vi "Main2.vi"() -> ()   [LabVIEW 2018]
uses:
  <vilib>/addons/zeromq/zmq_context.lvclass
  Communication Channel/Communication Channel.lvclass
  Channel Rep/Channel Rep.lvclass
  C:/Users/Denis/Desktop/communication-manager/communication-manager/Communication Channel/Communication Channel.lvclass
  Channel Req/Channel Req.lvclass
  Channel Pub/Channel Pub.lvclass
  Channel Sub/Channel Sub.lvclass
panel:
  in  "Channel Pub.lvclass":refnum<class "Channel Pub.lvclass">
  in  "Channel Sub.lvclass":refnum<class "Channel Sub.lvclass">
  in  "Channel Req.lvclass":refnum<class "Channel Req.lvclass">
  in  "Channel Rep.lvclass":refnum<class "Channel Rep.lvclass">
  out "context":refnum<class "zmq_context.lvclass">
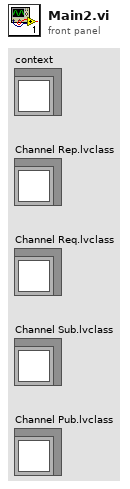
[diagram p1: front panel]
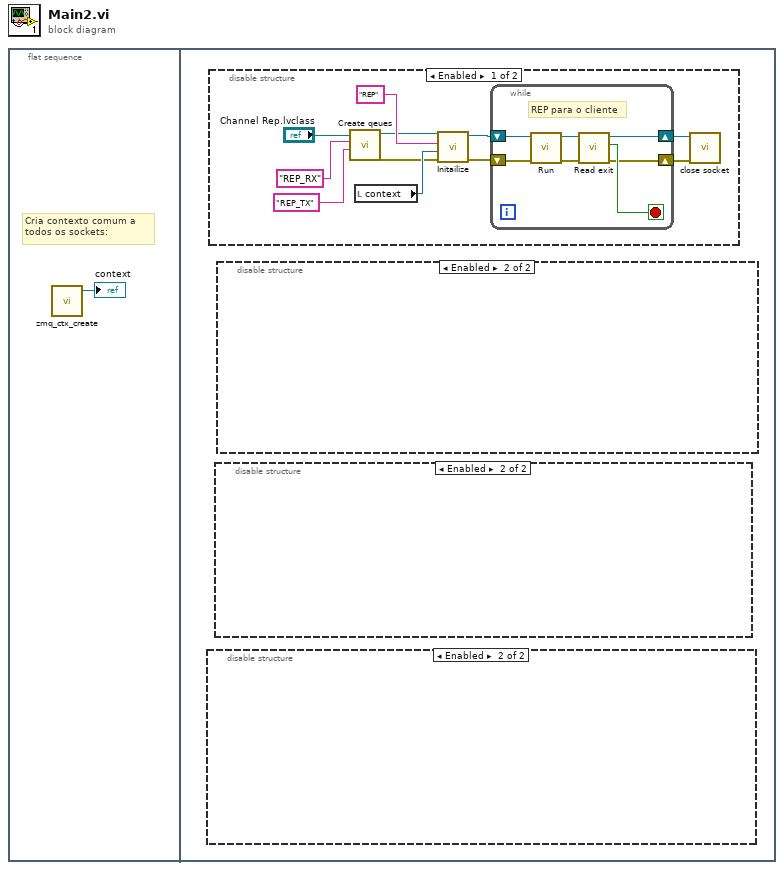
[diagram p0: block diagram]
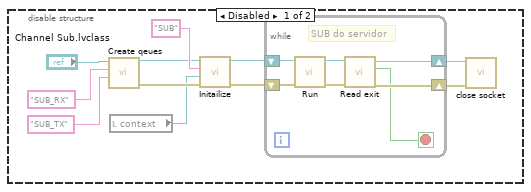
[diagram p2: hidden frame]
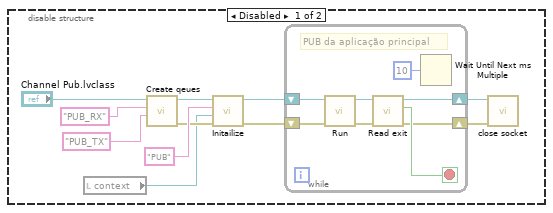
[diagram p3: hidden frame]
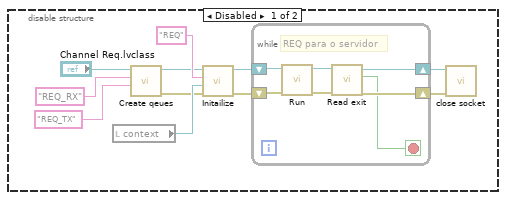
[diagram p4: hidden frame]
diagram:
  n1 = flat-sequence {
    frame #0 {
      # "Cria contexto comum a \ntodos os sockets:"
      n2 = call <vilib>:"zmq_ctx_create.vi"() -> ("context out"=→"context":refnum<class "zmq_context.lvclass">)  [unwired: 4 in, 1 out]
    }
    frame #1 {
      n3 = disable-structure shown="Enabled" {
        frame Disabled {
          n4 = local read "context"() -> (w20:refnum<class "zmq_context.lvclass">)
          n5 = call "Create qeues.vi"("name qeue Tx"="PUB_TX" ("name qeue Rx"), "name qeue Rx"="PUB_RX", "Communication Channel in"="Channel Pub.lvclass") -> ("error out"=w24:errorcluster, "Communication Channel out"=w25:refnum<class "Communication Channel.lvclass">)  [unwired: 7 in]
          n6 = call-dynamic "Initailize.vi"("error in (no error)"=w24, "zeromq.lvlib:ZeroMQ Context"=w20, "Name"="PUB", "Communication Channel in"=w25) -> ("error out"=w29:errorcluster, "Communication Channel out"=w30:refnum<class "Communication Channel.lvclass">)  [unwired: 6 in]
          n7 = while {
            shift-right: [w32] -> w27
            shift-left: w30 -> [w38]
            shift-right: [w33] -> w26
            shift-left: w29 -> [w37]
            stop <- w34 stop-if-true
            # "PUB da aplicação principal"
            n8 = call-dynamic "Run.vi"("error in (no error)"=w37, "Communication Channel in"=w38) -> ("error out"=w35:errorcluster, "Communication Channel out"=w36:refnum<class "Communication Channel.lvclass">)  [unwired: 8 in]
            n9 = call-dynamic "Read exit.vi"("error in (no error)"=w35, "Communication Channel in"=w36) -> ("error out"=w33:errorcluster, "exit"=w34:bool, "Communication Channel out"=w32:refnum<class "Communication Channel.lvclass">)  [unwired: 7 in]
            n10 = Wait Until Next ms Multiple(millisecond multiple=u32 10) -> ()  [unwired: 1 out]
          }
          n11 = call "close socket.vi"("error in (no error)"=w26, "Communication Channel in"=w27) -> ()  [unwired: 8 in, 2 out]
        }
        frame Enabled {
        }
      }
      n12 = disable-structure shown="Enabled" {
        frame Enabled {
          n13 = call "Create qeues.vi"("name qeue Tx"="REP_TX" ("name qeue Rx"), "name qeue Rx"="REP_RX", "Communication Channel in"="Channel Rep.lvclass") -> ("error out"=w61:errorcluster, "Communication Channel out"=w62:refnum<class "Communication Channel.lvclass">)  [unwired: 7 in]
          n14 = local read "context"() -> (w66:refnum<class "zmq_context.lvclass">)
          n15 = call-dynamic "Initailize.vi"("error in (no error)"=w61, "zeromq.lvlib:ZeroMQ Context"=w66, "Name"="REP", "Communication Channel in"=w62) -> ("error out"=w64:errorcluster, "Communication Channel out"=w65:refnum<class "Communication Channel.lvclass">)  [unwired: 6 in]
          n16 = while {
            shift-right: [w68] -> w57
            shift-left: w65 -> [w74]
            shift-right: [w69] -> w58
            shift-left: w64 -> [w73]
            stop <- w70 stop-if-true
            # "REP para o cliente"
            n17 = call-dynamic "Run.vi"("error in (no error)"=w73, "Communication Channel in"=w74) -> ("error out"=w71:errorcluster, "Communication Channel out"=w72:refnum<class "Communication Channel.lvclass">)  [unwired: 8 in]
            n18 = call-dynamic "Read exit.vi"("error in (no error)"=w71, "Communication Channel in"=w72) -> ("error out"=w69:errorcluster, "exit"=w70:bool, "Communication Channel out"=w68:refnum<class "Communication Channel.lvclass">)  [unwired: 7 in]
          }
          n19 = call "close socket.vi"("error in (no error)"=w58, "Communication Channel in"=w57) -> ()  [unwired: 8 in, 2 out]
        }
        frame Disabled {
        }
      }
      n20 = disable-structure shown="Enabled" {
        frame Disabled {
          n21 = call "Create qeues.vi"("name qeue Tx"="SUB_TX" ("name qeue Rx"), "name qeue Rx"="SUB_RX", "Communication Channel in"="Channel Sub.lvclass") -> ("error out"=w5:errorcluster, "Communication Channel out"=w6:refnum<class "Communication Channel.lvclass">)  [unwired: 7 in]
          n22 = local read "context"() -> (w2:refnum<class "zmq_context.lvclass">)
          n23 = call-dynamic "Initailize.vi"("error in (no error)"=w5, "zeromq.lvlib:ZeroMQ Context"=w2, "Name"="SUB", "Communication Channel in"=w6) -> ("error out"=w11:errorcluster, "Communication Channel out"=w12:refnum<class "Communication Channel.lvclass">)  [unwired: 6 in]
          n24 = while {
            shift-right: [w15] -> w9
            shift-left: w12 -> [w19]
            shift-right: [w14] -> w8
            shift-left: w11 -> [w18]
            stop <- w13 stop-if-true
            # "SUB do servidor"
            n25 = call-dynamic "Run.vi"("error in (no error)"=w18, "Communication Channel in"=w19) -> ("error out"=w16:errorcluster, "Communication Channel out"=w17:refnum<class "Communication Channel.lvclass">)  [unwired: 8 in]
            n26 = call-dynamic "Read exit.vi"("error in (no error)"=w16, "Communication Channel in"=w17) -> ("error out"=w14:errorcluster, "exit"=w13:bool, "Communication Channel out"=w15:refnum<class "Communication Channel.lvclass">)  [unwired: 7 in]
          }
          n27 = call "close socket.vi"("error in (no error)"=w8, "Communication Channel in"=w9) -> ()  [unwired: 8 in, 2 out]
        }
        frame Enabled {
        }
      }
      n28 = disable-structure shown="Enabled" {
        frame Disabled {
          n29 = local read "context"() -> (w48:refnum<class "zmq_context.lvclass">)
          n30 = call "Create qeues.vi"("name qeue Tx"="REQ_TX" ("name qeue Rx"), "name qeue Rx"="REQ_RX", "Communication Channel in"="Channel Req.lvclass") -> ("error out"=w43:errorcluster, "Communication Channel out"=w44:refnum<class "Communication Channel.lvclass">)  [unwired: 7 in]
          n31 = call-dynamic "Initailize.vi"("error in (no error)"=w43, "zeromq.lvlib:ZeroMQ Context"=w48, "Name"="REQ", "Communication Channel in"=w44) -> ("error out"=w46:errorcluster, "Communication Channel out"=w47:refnum<class "Communication Channel.lvclass">)  [unwired: 6 in]
          n32 = while {
            shift-right: [w52] -> w39
            shift-left: w47 -> [w56]
            shift-right: [w51] -> w40
            shift-left: w46 -> [w55]
            stop <- w50 stop-if-true
            # "REQ para o servidor"
            n33 = call-dynamic "Run.vi"("error in (no error)"=w55, "Communication Channel in"=w56) -> ("error out"=w53:errorcluster, "Communication Channel out"=w54:refnum<class "Communication Channel.lvclass">)  [unwired: 8 in]
            n34 = call-dynamic "Read exit.vi"("error in (no error)"=w53, "Communication Channel in"=w54) -> ("error out"=w51:errorcluster, "exit"=w50:bool, "Communication Channel out"=w52:refnum<class "Communication Channel.lvclass">)  [unwired: 7 in]
          }
          n35 = call "close socket.vi"("error in (no error)"=w40, "Communication Channel in"=w39) -> ()  [unwired: 8 in, 2 out]
        }
        frame Enabled {
        }
      }
    }
  }
